vi "Paused Next State.vi"(8 "error in":errorcluster, 11 "Command":T2) -> (0 "error out":errorcluster, 3 "State":T1)   [LabVIEW 2013, in "synchronous engine runtime.lvclass"]
uses:
  synchronous engine runtime.lvclass
  Commands.ctl
  Engine Runtime/Execution States.ctl
  Engine Runtime/Engine Runtime Interface.lvclass
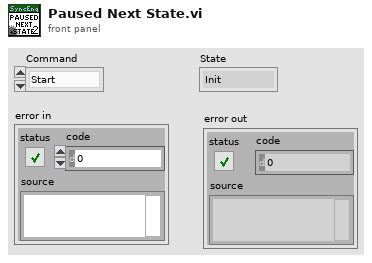
[diagram p1: front panel]
types:
  T1 = typedef "Engine Runtime Interface.lvclass/Execution States.ctl" = enum16{"Init", "Pre-Operational", "Safe-Operational", "Operational", "Stopped"}
  T2 = typedef "synchronous engine runtime.lvclass/Commands.ctl" = enum16{"Start", "Pause", "Safe State", "Normal", "Stop", "Shutdown"}
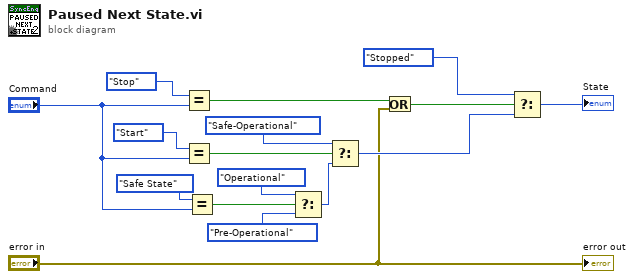
[diagram p0: block diagram]
diagram:
  n1 = Equal?(x=Commands."Stop" ("Commands"), y="Command") -> (x = y?=w11:bool)
  n2 = Equal?(x=Commands."Start" ("Commands"), y="Command") -> (x = y?=w8:bool)
  n3 = Equal?(x=Commands."Safe State" ("Commands"), y="Command") -> (x = y?=w4:bool)
  n4 = Select(t=Execution_States."Operational", s=w4, f=Execution_States."Pre-Operational" ("States")) -> (s? t:f=w2:T1)
  n5 = Select(t=Execution_States."Safe-Operational" ("States"), s=w8, f=w2) -> (s? t:f=w10:T1)
  n6 = Or(x=w11, y="error in") -> (x .or. y?=w12:bool)
  n7 = Select(t=Execution_States."Stopped" ("States"), s=w12, f=w10) -> (s? t:f=→"State":T1)
  "error out" <- "error in"
